vi "GFITS_GetExtmap.vi"(10 "num_ext":i32) -> (1 "num extensions":i32, 2 "strout":string)   [LabVIEW 2016]
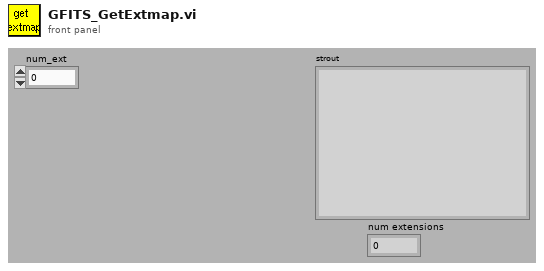
[diagram p1: front panel]
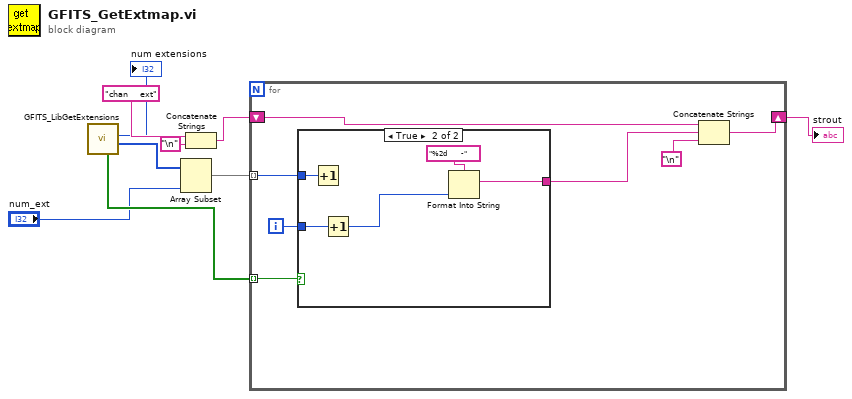
[diagram p0: block diagram]
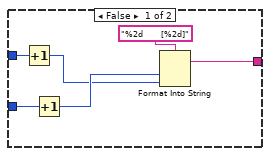
[diagram p2: hidden frame]
diagram:
  n1 = call "GFITS_LibGetExtensions.vi"() -> ("array out"=w9:i32[], "num extensions"=→"num extensions":i32, "discard"=w7:bool[])  [unwired: 2 in, 7 out]
  n2 = Array Subset(array=w9, length="num_ext") -> (w8:i32[])  [unwired: 1 in]
  n3 = Concatenate Strings("chan    ext", "\n") -> (w3:string)
  n4 = for {
    tunnel: w8 -> [w16] mode=indexing
    shift-right: [w13] -> w2
    shift-left: w3 -> [w15]
    tunnel: w7 -> [w10] mode=indexing
    i -> [w11]
    n5 = case shown="True" w10 {
      tunnel: w16 -> [w21 w26]
      tunnel: [w20 w25] -> w12
      tunnel: w11 -> [w19 w24]
      frame False {
        n6 = Increment(x=w21) -> (x+1=w17:i32)
        n7 = Increment(x=w19) -> (x+1=w18:i32)
        n8 = Format Into String(format string="%2d      [%2d]", w18, w17) -> (resulting string=w20:string)  [unwired: 2 in, 1 out]
      }
      frame True {
        n9 = Increment(x=w26) -> ()  [unwired: 1 out]
        n10 = Increment(x=w24) -> (x+1=w23:i32)
        n11 = Format Into String(format string="%2d       -", w23) -> (resulting string=w25:string)  [unwired: 2 in, 1 out]
      }
    }
    n12 = Concatenate Strings(w15, w12, "\n") -> (w13:string)
  }
  "strout" <- w2
